vi "cor_diferenca.vi"() -> ()   [LabVIEW 2016]
uses:
  <vilib>/NXT/Subs/LVHSConnector.ctl
  <vilib>/NXT/LegoClasses/BrickReference/BrickReference.lvclass
  parametros.ctl
  <vilib>/NXT/Block Support/NXT_InputPort.ctl
  <vilib>/NXT/Subs/ColorSensorColors.ctl
  <vilib>/NXT/Dual Mode Library/prims/sortArray/sortArray_float.vi
panel:
  out "Cor":T1
  in  "Parâmetros Ini":T2={"Gyro Port"=0, "Sensor - Left"=3, "Sensor - Right"=2, "     Color \nSensor Port"=1, "Kp Front"=0.5, "Motor speed"=-15, "Distance to street"=0.0, "Motor speed turns"=16, "Kp Curvas"=0.0} {"Kp Front" format="%.3f"; "Color \nSensor Port" items=["Port 1", "Port 2", "Port 3", "Port 4"]; "Sensor - Right" items=["Port 1", "Port 2", "Port 3", "Port 4"]; "Sensor - Left" items=["Port 1", "Port 2", "Port 3", "Port 4"]; "Gyro Port" items=["Port 1", "Port 2", "Port 3", "Port 4"]}
  out "NXT/EV3 2":T4
  in  "NXT/EV3":T4
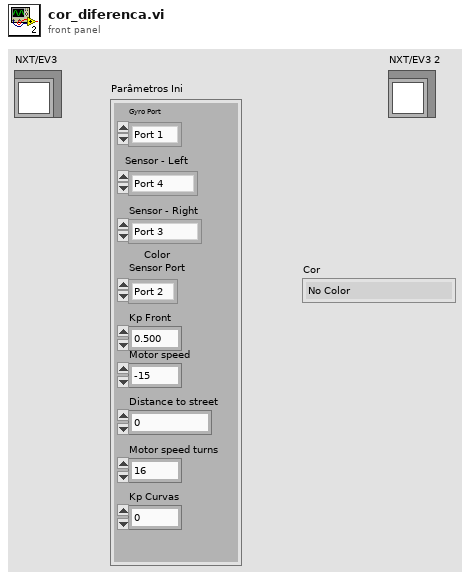
[diagram p1: front panel]
types:
  T1 = typedef "ColorSensorColors.ctl" = enum16{"No Color", "Black", "Blue", "Green", "Yellow", "Red", "White", "Brown"}
  T2 = typedef "parametros.ctl" = cluster{"Gyro Port":T3, "Sensor - Left":T3, "Sensor - Right":T3, "     Color \nSensor Port":T3, "Kp Front":dbl, "Motor speed":i32, "Distance to street":dbl, "Motor speed turns":i32, "Kp Curvas":dbl}
  T3 = typedef "NXT_InputPort.ctl" = u32
  T4 = typedef "LVHSConnector.ctl" = refnum<class "BrickReference.lvclass">
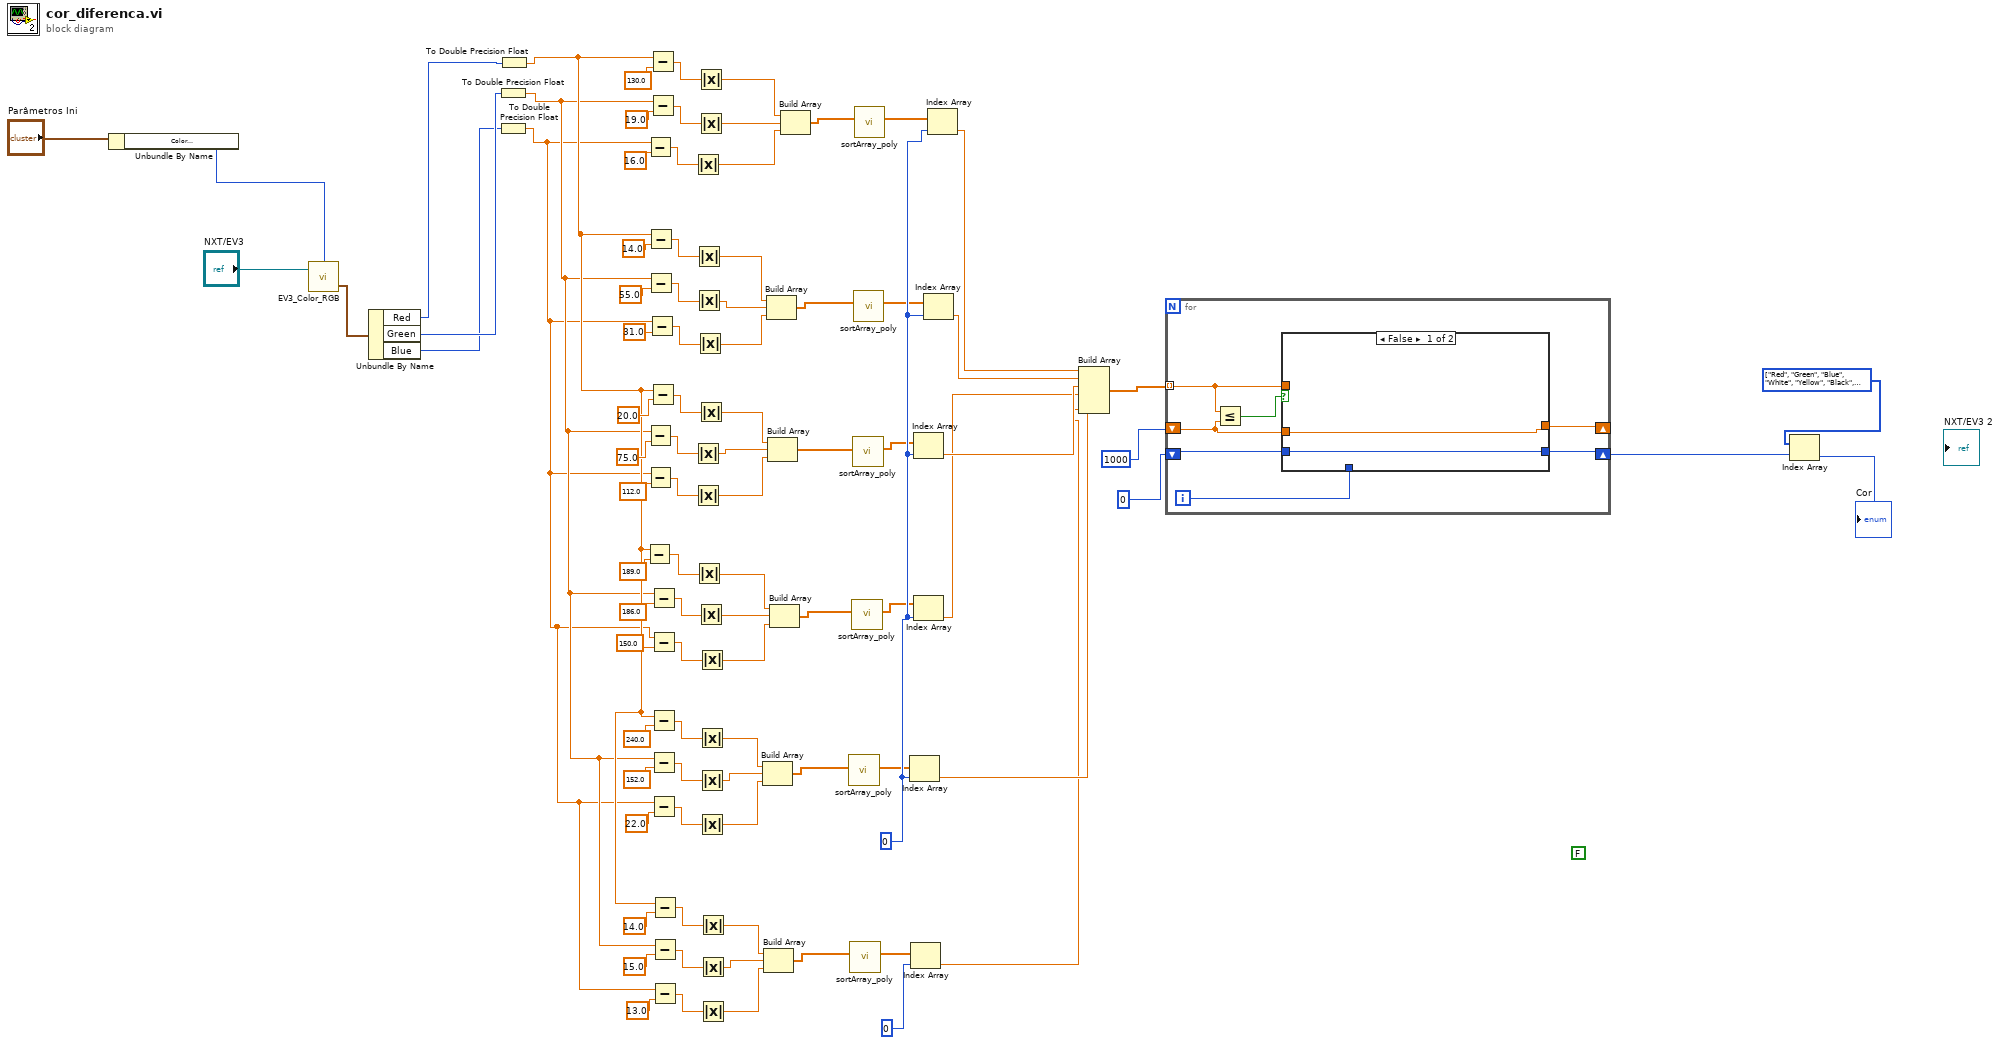
[diagram p0: block diagram]
diagram:
  w3 = T1[] [enum."Red", enum."Green", enum."Blue", enum."White", enum."Yellow", enum."Black", enum."White", enum."Blue"] items=["No Color", "Black", "Blue", "Green", "Yellow", "Red", "White", "Brown"]
  (unwired) FALSE
  w35 = 0 ("index")
  n1 = Unbundle By Name("Parâmetros Ini") -> ("Color \nSensor Port"=w20:T3)
  n2 = call <vilib>:"EV3_Color_RGB.vi"("NXT/EV3"="NXT/EV3", "Port (Port 1)"=w20) -> ("RGB Color"=w89:cluster{"Red":u8, "Green":u8, "Blue":u8})  [unwired: 1 in, 1 out]
  n3 = Unbundle By Name(w89) -> ("Red"=w73:u8, "Green"=w72:u8, "Blue"=w71:u8)
  n4 = To Double Precision Float(number=w72) -> (double precision float=w6:dbl)
  n5 = To Double Precision Float(number=w71) -> (double precision float=w5:dbl)
  n6 = To Double Precision Float(number=w73) -> (double precision float=w7:dbl)
  n7 = Subtract(x=w7, y=189.0) -> (x-y=w79:dbl)
  n8 = Subtract(x=w5, y=16.0) -> (x-y=w86:dbl)
  n9 = Subtract(x=w6, y=75.0) -> (x-y=w81:dbl)
  n10 = Subtract(x=w5, y=112.0) -> (x-y=w80:dbl)
  n11 = Subtract(x=w7, y=14.0) -> (x-y=w85:dbl)
  n12 = Subtract(x=w6, y=55.0) -> (x-y=w84:dbl)
  n13 = Subtract(x=w5, y=31.0) -> (x-y=w83:dbl)
  n14 = Subtract(x=w7, y=130.0) -> (x-y=w88:dbl)
  n15 = Subtract(x=w6, y=19.0) -> (x-y=w87:dbl)
  n16 = Subtract(x=w7, y=20.0) -> (x-y=w82:dbl)
  n17 = Subtract(x=w6, y=186.0) -> (x-y=w78:dbl)
  n18 = Subtract(x=w5, y=150.0) -> (x-y=w77:dbl)
  n19 = Subtract(x=w7, y=240.0) -> (x-y=w76:dbl)
  n20 = Subtract(x=w6, y=152.0) -> (x-y=w75:dbl)
  n21 = Subtract(x=w5, y=22.0) -> (x-y=w74:dbl)
  n22 = Subtract(x=w7, y=14.0) -> (x-y=w19:dbl)
  n23 = Subtract(x=w6, y=15.0) -> (x-y=w18:dbl)
  n24 = Subtract(x=w5, y=13.0) -> (x-y=w17:dbl)
  n25 = Absolute Value(x=w86) -> (abs(x)=w53:dbl)
  n26 = Absolute Value(x=w81) -> (abs(x)=w48:dbl)
  n27 = Absolute Value(x=w80) -> (abs(x)=w47:dbl)
  n28 = Absolute Value(x=w85) -> (abs(x)=w52:dbl)
  n29 = Absolute Value(x=w84) -> (abs(x)=w51:dbl)
  n30 = Absolute Value(x=w79) -> (abs(x)=w46:dbl)
  n31 = Absolute Value(x=w83) -> (abs(x)=w50:dbl)
  n32 = Absolute Value(x=w88) -> (abs(x)=w55:dbl)
  n33 = Absolute Value(x=w87) -> (abs(x)=w54:dbl)
  n34 = Absolute Value(x=w82) -> (abs(x)=w49:dbl)
  n35 = Absolute Value(x=w78) -> (abs(x)=w45:dbl)
  n36 = Absolute Value(x=w77) -> (abs(x)=w44:dbl)
  n37 = Absolute Value(x=w76) -> (abs(x)=w43:dbl)
  n38 = Absolute Value(x=w75) -> (abs(x)=w42:dbl)
  n39 = Absolute Value(x=w74) -> (abs(x)=w41:dbl)
  n40 = Absolute Value(x=w19) -> (abs(x)=w13:dbl)
  n41 = Absolute Value(x=w18) -> (abs(x)=w12:dbl)
  n42 = Absolute Value(x=w17) -> (abs(x)=w11:dbl)
  n43 = Build Array(w43, w42, w41) -> (w36:dbl[])
  n44 = Build Array(w13, w12, w11) -> (w10:dbl[])
  n45 = Build Array(w52, w51, w50) -> (w39:dbl[])
  n46 = Build Array(w49, w48, w47) -> (w38:dbl[])
  n47 = Build Array(w46, w45, w44) -> (w37:dbl[])
  n48 = Build Array(w55, w54, w53) -> (w40:dbl[])
  n49 = call-poly <vilib>:"sortArray_poly.vi"("array"=w36) -> ("sorted array"=w30:dbl[])  [unwired: 10 in]
  n50 = call-poly <vilib>:"sortArray_poly.vi"("array"=w10) -> ("sorted array"=w8:dbl[])  [unwired: 10 in]
  n51 = call-poly <vilib>:"sortArray_poly.vi"("array"=w37) -> ("sorted array"=w31:dbl[])  [unwired: 10 in]
  n52 = call-poly <vilib>:"sortArray_poly.vi"("array"=w38) -> ("sorted array"=w32:dbl[])  [unwired: 10 in]
  n53 = call-poly <vilib>:"sortArray_poly.vi"("array"=w39) -> ("sorted array"=w33:dbl[])  [unwired: 10 in]
  n54 = call-poly <vilib>:"sortArray_poly.vi"("array"=w40) -> ("sorted array"=w34:dbl[])  [unwired: 10 in]
  n55 = Index Array(array=w30, index=w35) -> (element=w25:dbl)
  n56 = Index Array(array=w8, index=0) -> (element=w4:dbl)
  n57 = Index Array(array=w32, index=w35) -> (element=w27:dbl)
  n58 = Index Array(array=w31, index=w35) -> (element=w26:dbl)
  n59 = Index Array(array=w33, index=w35) -> (element=w28:dbl)
  n60 = Index Array(array=w34, index=w35) -> (element=w29:dbl)
  n61 = Build Array(w29, w28, w27, w26, w25, w4) -> (w23:dbl[])
  n62 = for {
    tunnel: w23 -> [w95] mode=indexing
    shift-right: [w96] -> _
    shift-left: 1000 -> [w94]
    shift-right: [w92] -> w2
    shift-left: 0 -> [w91]
    i -> [w93]
    n63 = Less Or Equal?(x=w95, y=w94) -> (x <= y?=w97:bool)
    n64 = case shown="False" w97 {
      tunnel: [w99 w101] -> w96
      tunnel: w95 -> [_ w101]
      tunnel: w94 -> [w99 _]
      tunnel: w93 -> [_ w100]
      tunnel: [w98 w100] -> w92
      tunnel: w91 -> [w98 _]
      frame False {
      }
      frame True {
      }
    }
  }
  n65 = Index Array(array=w3, index=w2) -> (element=→"Cor":T1)
